vi "Shift LSB.vi"(1 "Binary Data In":u32, 3 "Error In":errorcluster) -> (8 "Binary Service Binary out":u32, 10 "Error Out":errorcluster)   [LabVIEW 2016]
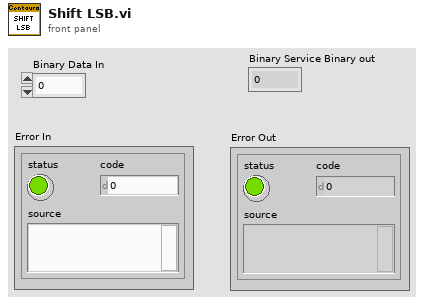
[diagram p1: front panel]
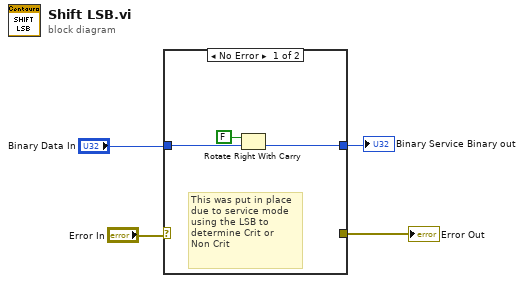
[diagram p0: block diagram]
diagram:
  n1 = case shown="No Error" "Error In" {
    selector: "Error In" -> [_ w8]
    tunnel: [w6 w9] -> w4
    tunnel: "Binary Data In" -> [w5 w9]
    tunnel: [_ w8] -> w1
    frame No Error {
      # "This was put in place\ndue to service mode\nusing the LSB to\ndetermine Crit or \nNon Crit"
      n2 = Rotate Right With Carry(2:w5, 3:FALSE ("Standalone?")) -> (0:w6:u32)  [unwired: 1 out]
    }
    frame Error {
    }
  }
  "Binary Service Binary out" <- w4
  "Error Out" <- w1
